vi "Reset.vi"(8 "error in (no error)":errorcluster, 11 "Iterate in":refnum<class "Abs_Waveform.lvclass">) -> (0 "error out":errorcluster, 3 "Iterate out":refnum<class "Abs_Waveform.lvclass">)   [LabVIEW 2021, in "Abs_Waveform.lvclass"]
uses:
  Abs_Waveform.lvclass
  Abs_Waveform.lvclass/Abs_Waveform.ctl
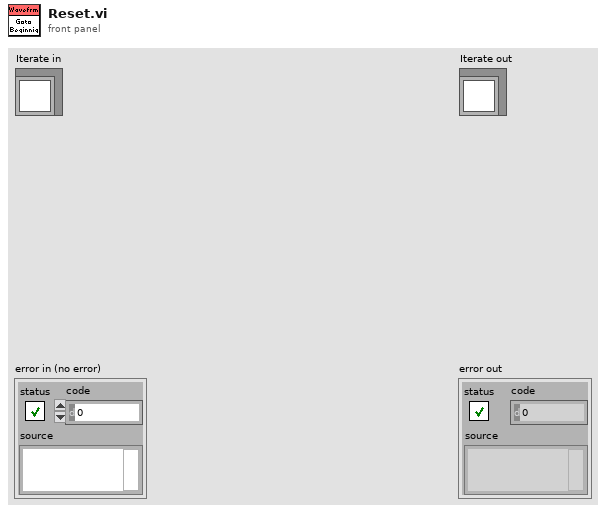
[diagram p1: front panel]
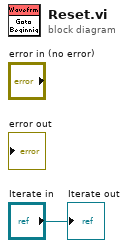
[diagram p0: block diagram]
diagram:
  "Iterate out" <- "Iterate in"
